vi "Get Indexes of Multiple Wheels from Names.vi"(8 "error in (no error)":errorcluster, 10 "wheel names":string[](array[string]), 11 "steering frame in":refnum<class "NI_Robotics_Steering Frame.lvclass">) -> (0 "error out":errorcluster, 1 "found?":bool[](array[boolean]), 2 "indexes":i32[](array[numeric]), 3 "steering frame out":refnum<class "NI_Robotics_Steering Frame.lvclass">)   [LabVIEW 2017, in "NI_Robotics_Steering Frame.lvclass"]
uses:
  <vilib>/robotics/Steering/Steering Frame/NI_Robotics_Steering Frame.lvclass
  <vilib>/robotics/Steering/Steering Frame/NI_Robotics_Steering Frame.lvclass/NI_Robotics_Steering Frame.ctl
  <vilib>/robotics/Steering/Wheel/NI_Robotics_Wheel.lvclass/NI_Robotics_Wheel.ctl
  <vilib>/robotics/Steering/Wheel/NI_Robotics_Wheel.lvclass
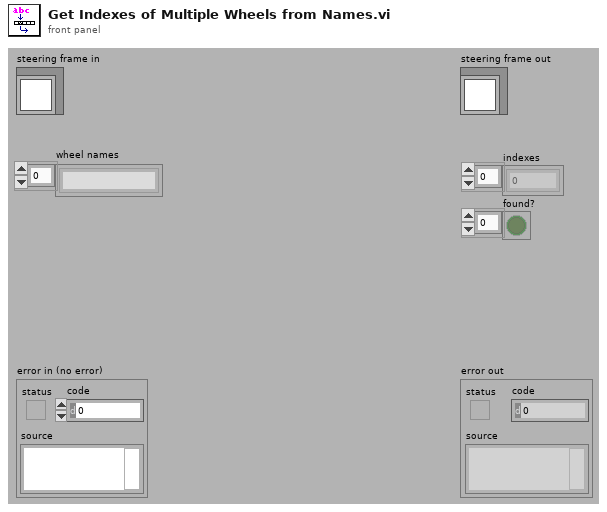
[diagram p1: front panel]
types:
  T1 = typedef "NI_Robotics_Steering Frame.lvclass/Wheel Orientation.ctl" = cluster{"wheel":refnum<class "NI_Robotics_Wheel.lvclass">, "x position":dbl, "y position":dbl, "frame angle (rad)":dbl}
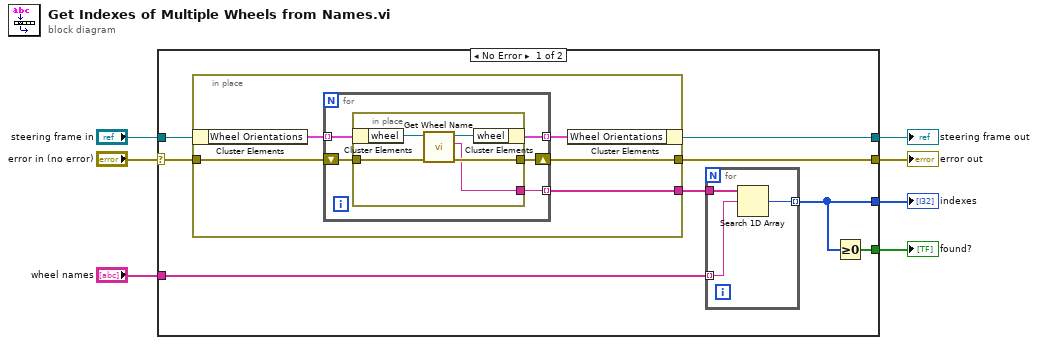
[diagram p0: block diagram]
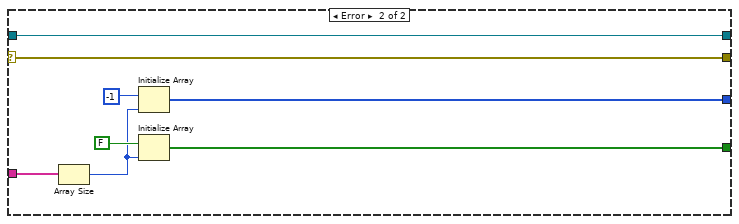
[diagram p2: hidden frame]
diagram:
  n1 = case shown="No Error" "error in (no error)" {
    selector: "error in (no error)" -> [w13 w41]
    tunnel: [w12 w41] -> w6
    tunnel: [w14 w40] -> w4
    tunnel: "steering frame in" -> [w15 w40]
    tunnel: "wheel names" -> [w11 w38]
    tunnel: [w8 w37] -> w2
    tunnel: [w9 w34] -> w3
    frame No Error {
      n2 = in-place {
        in-place-border: w13 -> [w22]
        in-place-border: [w20] -> w12
        in-place-border: [w19] -> w10
        n3 = in-place-cluster #1(w15) -> ("Wheel Orientations"=w23:T1[])
        n4 = for {
          tunnel: w23 -> [w28] mode=indexing
          shift-right: [w26] -> w20
          shift-left: w22 -> [w27]
          tunnel: [w25] -> w21 mode=indexing
          tunnel: [w24] -> w19 mode=indexing
          n5 = in-place {
            in-place-border: [w31] -> w26
            in-place-border: [w30] -> w24
            in-place-border: w27 -> [w29]
            n6 = in-place-cluster #2(w28) -> ("wheel"=w33:refnum<class "NI_Robotics_Wheel.lvclass">)
            n7 = call <vilib>:"Get Wheel Name.vi"("error in (no error)"=w29, "wheel in"=w33) -> ("error out"=w31:errorcluster, "wheel name"=w30:string, "wheel out"=w32:refnum<class "NI_Robotics_Wheel.lvclass">)  [unwired: 7 in]
            n8 = in-place-cluster #2("wheel"=w32) -> (w25:T1)
          }
        }
        n9 = in-place-cluster #1("Wheel Orientations"=w21) -> (w14:refnum<class "NI_Robotics_Steering Frame.lvclass">)
      }
      n10 = for {
        tunnel: w11 -> [w17] mode=indexing
        tunnel: w10 -> [w18]
        tunnel: [w16] -> w9 mode=indexing
        n11 = Search 1D Array(1D array=w18, element=w17) -> (index of element=w16:i32)  [unwired: 1 in]
      }
      n12 = Greater Or Equal To 0?(x=w9) -> (x >= 0?=w8:bool[])
    }
    frame Error {
      n13 = Array Size(array=w38) -> (size(s)=w36:i32)
      n14 = Initialize Array(-1 ("size(s)"), w36) -> (w34:i32[])
      n15 = Initialize Array(FALSE, w36) -> (w37:bool[])
    }
  }
  "error out" <- w6
  "steering frame out" <- w4
  "indexes" <- w3
  "found?" <- w2
